vi "GFITS_GeomKeyPreview.vi"(8 "error in (no error)":errorcluster, 10 "args":string, 11 "Database RefNum in":T1) -> (0 "error out":errorcluster, 2 "preview":string)   [LabVIEW 2016]
uses:
  DBSHAND/private/vis/DatabaseHand_RefNum.ctl
  DBSHAND/private/vis/DatabaseHand_Element_Get(string).vi
  DBSHAND/private/vis/DatabaseHand_Element_Get(bool).vi
  GFITS_Gbls.vi
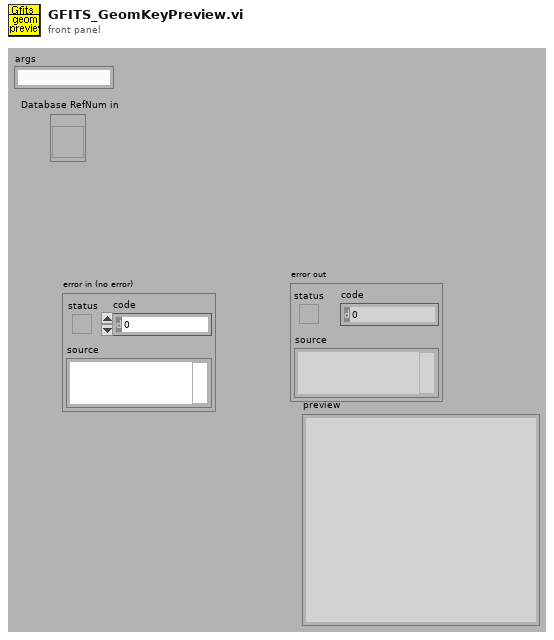
[diagram p1: front panel]
types:
  T1 = typedef "DatabaseHand_RefNum.ctl" = refnum<vi>
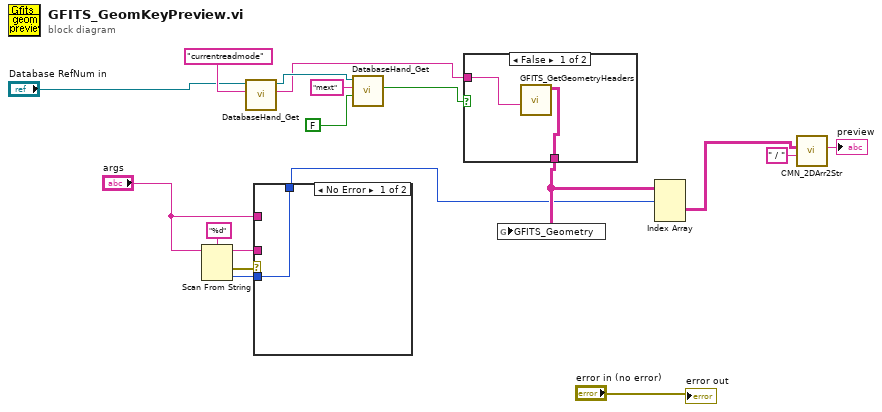
[diagram p0: block diagram]
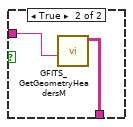
[diagram p2: hidden frame]
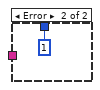
[diagram p3: hidden frame]
diagram:
  n1 = Scan From String(format string="%d", input string="args") -> (remaining string=w13:string, error out=w15:errorcluster, output 1=w14:i32)  [unwired: 2 in, 2 out]
  n2 = call-poly "DatabaseHand_Get.vi"("name"="currentreadmode", "Database RefNum in"="Database RefNum in") -> ("value"=w5:string, "Database RefNum out"=w10:T1)  [unwired: 3 in, 5 out]
  n3 = case shown="No Error" w15 {
    tunnel: w14 -> [w19 _]
    tunnel: w13 -> [_ _]
    tunnel: [w19 1] -> w3
    tunnel: "args" -> [_ _]
    frame No Error {
    }
    frame Error {
    }
  }
  n4 = call-poly "DatabaseHand_Get.vi"("default value"=FALSE, "name"="mext", "Database RefNum in"=w10) -> ("value"=w6:bool)  [unwired: 2 in, 6 out]
  n5 = case shown="False" w6 {
    tunnel: w5 -> [w21 w24]
    tunnel: [w22 w23] -> w4
    frame False {
      n6 = call "GFITS_GetGeometryHeaders.vi"("readmode"=w21) -> ("Keywords out"=w22:string[][][])  [unwired: 10 out]
    }
    frame True {
      n7 = call "GFITS_GetGeometryHeadersM.vi"("readmode"=w24) -> ("Keywords out"=w23:string[][][])  [unwired: 10 out]
    }
  }
  n8 = global write "GFITS_Gbls.vi" "GFITS_Geometry"(w4) -> ()
  n9 = Index Array(array=w4, index (dim 0)=w3) -> (element=w2:string[][])  [unwired: 2 in]
  n10 = call "CMN_2DArr2Str.vi"("separator"=" / ", "array in"=w2) -> ("string out"=→"preview":string)  [unwired: 9 out]
  "error out" <- "error in (no error)"
